vi "SetPort.vi"(8 "error in (no error)":errorcluster, 9 "Value":u8, 10 "Port":u8, 11 "NXP LPCXpresso54608 in":refnum<class "NXP LPCXpresso54608.lvclass">) -> (0 "error out":errorcluster, 3 "NXP LPCXpresso54608 out":refnum<class "NXP LPCXpresso54608.lvclass">)   [LabVIEW 2020, in "NXP LPCXpresso54608.lvclass"]
doc: "Set a value on a port on the target device."
uses:
  NXP LPCXpresso54608.lvclass
  MCU/MCU.lvclass
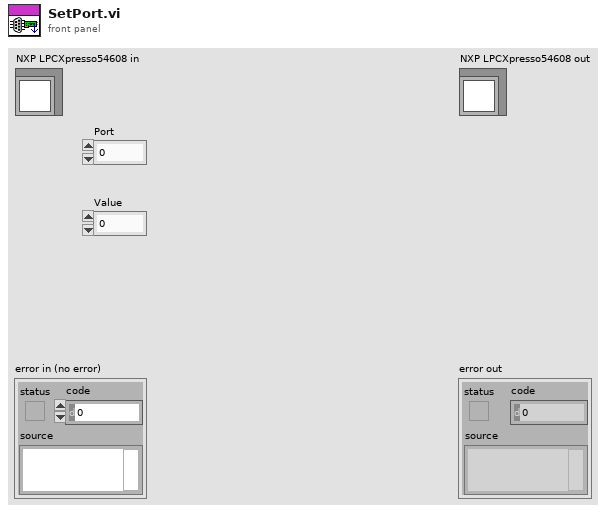
[diagram p1: front panel]
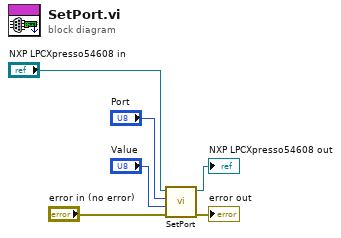
[diagram p0: block diagram]
diagram:
  n1 = call-parent "SetPort.vi"("error in (no error)"="error in (no error)", "Value"="Value", "Port"="Port", "MCU in"="NXP LPCXpresso54608 in") -> ("error out"=→"error out":errorcluster, "MCU out"=→"NXP LPCXpresso54608 out":refnum<class "NXP LPCXpresso54608.lvclass">)  [unwired: 6 in]
